vi "DoHandshake.vi"(6 "Additional Return headers (none)":T1[](array[typedef]), 8 "error in (no error)":errorcluster, 9 "timeout ms (5000)":i32=5000, 10 "Supported Protocols (any)":string[](array[string]), 11 "TCP Connection in":refnum<k5>) -> (0 "error out":errorcluster, 1 "Request URI":string, 2 "Client Headers":variant, 3 "WebSocket Server out":refnum<class "WebSocket Server.lvclass">)   [LabVIEW 2021, in "WebSockets.lvlib"]
doc: "**Deprecated - please use the new WebSocket.lvclass VIs instead. VI is retained for backwards compatibility.**\n\nPerforms the WebSockets HTTP handshaking on the new TCP connection. The client sends HTTP headers and the server must reply with a correctly formed HTTP response. The VI handles an incoming WS-Protocol and will return it in the response headers if it matches the supported protocols input. Additional HTTP headers can also be returned.\nWebSockets 2.0.1.40\nSam Sharp - MediaMongrels Ltd\nCopyright (c) 2019, MediaMongrels Ltd"
uses:
  WebSockets.lvlib
  WebSocket Server/WebSocket Server.lvclass
  C:/my_projects/projects/Algorithms/Labview/21/WebSockets/WebSockets/WebSocket/WebSocket.lvclass
  WebSocket/Headers.ctl
  WebSocket/WebSocket.lvclass/WebSocket.ctl
  WebSocket Server/WebSocket Server.lvclass/WebSocket Server.ctl
  WebSocket/Write Protocols.vi
  WebSocket/Read Return Headers.vi
  WebSocket Server/Read Request URI.vi
  Sockets/VISA TCP Socket/VISA TCP.lvclass
  C:/my_projects/projects/Algorithms/Labview/21/WebSockets/Sockets/Socket/Socket.lvclass
  WebSocket/Write Send Headers.vi
  WebSocket/WebSocket.lvclass
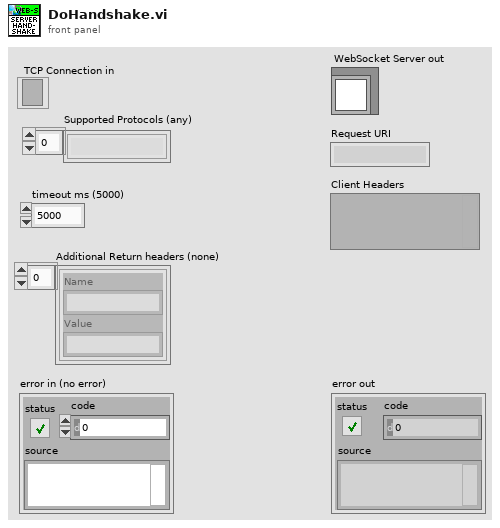
[diagram p1: front panel]
types:
  T1 = typedef "WebSockets.lvlib/WebSocket.lvclass/Headers.ctl" = cluster{"Name":string, "Value":string}
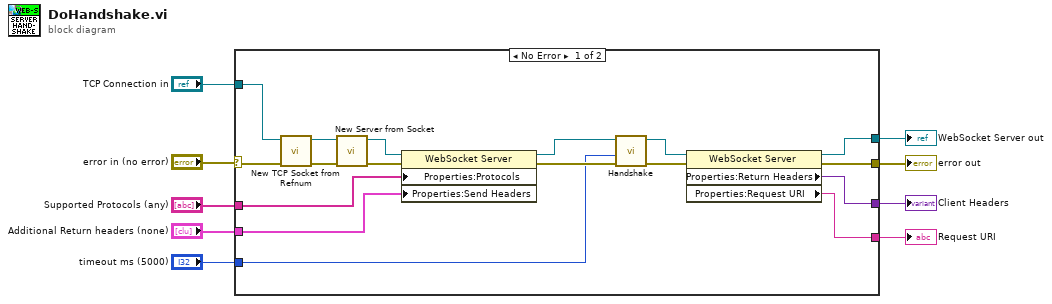
[diagram p0: block diagram]
diagram:
  n1 = case shown="No Error" "error in (no error)" {
    selector: "error in (no error)" -> [w15 w27]
    tunnel: [w19 _] -> w9
    tunnel: "TCP Connection in" -> [w14 _]
    tunnel: [w21 w27] -> w6
    tunnel: "timeout ms (5000)" -> [w23 _]
    tunnel: [w18 _] -> w4
    tunnel: [w16 _] -> w3
    tunnel: "Supported Protocols (any)" -> [w17 _]
    tunnel: "Additional Return headers (none)" -> [w22 _]
    frame No Error {
      n2 = call "New TCP Socket from Refnum.vi"("error in (no error)"=w15, "TCP Network Connection Refnum"=w14) -> ("error out"=w13:errorcluster, "VISA TCP out"=w12:refnum<class "VISA TCP.lvclass">)  [unwired: 8 in]
      n3 = call "New Server from Socket.vi"("error in (no error)"=w13, "Socket"=w12) -> ("error out"=w10:errorcluster, "WebSocket Server out"=w11:refnum<class "WebSocket Server.lvclass">)  [unwired: 8 in]
      n4 = property class="WebSocket Server"(reference=w11, error in=w10, "Properties:Protocols"=w17, "Properties:Send Headers"=w22) -> (reference out=w25:refnum<class "WebSocket Server.lvclass">, error out=w26:errorcluster)
      n5 = call-dynamic "Handshake.vi"("error in (no error)"=w26, "timeout ms (5000)"=w23, "WebSocket Connection in"=w25) -> ("error out"=w24:errorcluster, "WebSocket Connection out"=w20:refnum<class "WebSocket Server.lvclass">)  [unwired: 7 in]
      n6 = property class="WebSocket Server"(reference=w20, error in=w24) -> (reference out=w19:refnum<class "WebSocket Server.lvclass">, error out=w21:errorcluster, "Properties:Return Headers"=w18:variant, "Properties:Request URI"=w16:string)
    }
    frame Error {
    }
  }
  "WebSocket Server out" <- w9
  "error out" <- w6
  "Client Headers" <- w4
  "Request URI" <- w3
